vi "DAQ6363_WaitPulseDone.vi"(4 "Timeout(ms)":u32=20000, 6 "HaltRef":refnum<vi>, 8 "error in (no error)":errorcluster caption="entrée d'erreur (pas d'erreur)", 11 "TaskIn":refnum<k21>) -> (0 "error out":errorcluster caption="sortie d'erreur", 3 "TaskOut":refnum<k21>)   [LabVIEW 2019]
uses:
  <userlib>/GenProg/ReadValByRefBool.vi
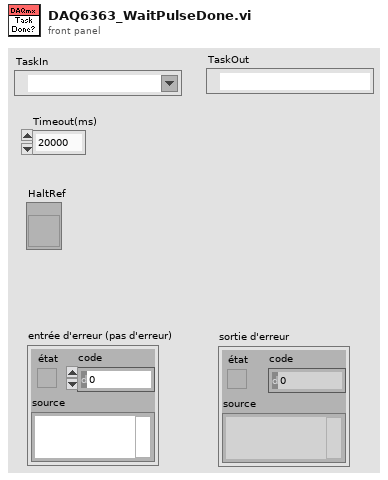
[diagram p1: front panel]
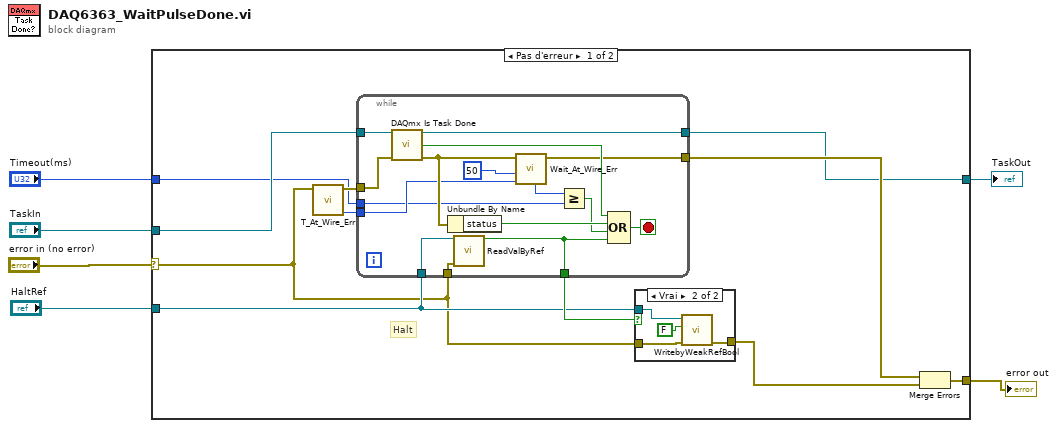
[diagram p0: block diagram]
diagram:
  n1 = case shown="Pas d'erreur" "error in (no error)" {
    selector: "error in (no error)" -> [w10 w40]
    tunnel: [w15 w40] -> w5
    tunnel: "TaskIn" -> [w13 w39]
    tunnel: "HaltRef" -> [w16 _]
    tunnel: [w11 w39] -> w2
    tunnel: "Timeout(ms)" -> [w7 _]
    frame No Error {
      # "Halt"
      n2 = call <userlib>:"T_At_Wire_Err.vi"("error in (no error)"=w10) -> ("Clock(ms)"=w8:u32, "error out"=w9:errorcluster)  [unwired: 8 in, 1 out]
      n3 = while {
        tunnel: w13 -> [w38]
        tunnel: w9 -> [w37]
        tunnel: [w27] -> w12
        tunnel: [w35] -> w11
        tunnel: w16 -> [w32]
        tunnel: w10 -> [w31]
        tunnel: [w30] -> w17
        tunnel: w8 -> [w26]
        tunnel: w7 -> [w24]
        stop <- w36 stop-if-true
        n4 = call <vilib>:"DAQmx Is Task Done.vi"("task/channels in"=w38, "error in"=w37) -> ("task out"=w35:refnum<k21>, "task done?"=w33:bool, "error out"=w29:errorcluster)  [unwired: 11 in]
        n5 = Unbundle By Name(w29) -> ("status"=w34:bool)
        n6 = call-poly <userlib>:"ReadValByRef.vi"("Control Ref"=w32, "error in"=w31) -> ("Valeur"=w30:bool)  [unwired: 12 in, 1 out]
        n7 = call <userlib>:"Wait_At_Wire_Err.vi"("InitClock(ms)"=w26, "Wait (ms)"=u32 50, "error in (no error)"=w29) -> ("error out"=w27:errorcluster, "Delta(ms)"=w25:u32)  [unwired: 6 in, 1 out]
        n8 = Greater Or Equal?(x=w25, y=w24) -> (x >= y?=w23:bool)
        n9 = Compound Arithmetic op=OR(w33, w34, w23, w30) -> (w36:bool)
      }
      n10 = case shown="Vrai" w17 {
        tunnel: w16 -> [_ w22]
        tunnel: [w18 w20] -> w14
        tunnel: w10 -> [w18 w19]
        frame False {
        }
        frame True {
          n11 = call <userlib>:"WritebyWeakRefBool.vi"("error in"=w19, "Valeur"=FALSE, "Control Ref"=w22) -> ("error out"=w20:errorcluster)  [unwired: 8 in]
        }
      }
      n12 = Merge Errors(w12, w14) -> (w15:errorcluster)
    }
    frame Error {
    }
  }
  "error out" <- w5
  "TaskOut" <- w2
